vi "Delete Pulse.vi"(8 "error in (no error)":errorcluster, 10 "Shot":i32, 11 "Tree in":refnum<class "Tree.lvclass">) -> (0 "error out":errorcluster, 3 "Tree out":refnum<class "Tree.lvclass">)   [LabVIEW 2013, in "MDSplus.lvlib" / "Tree.lvclass"]
doc: "Delete a pulse file."
uses:
  <vilib>/MDSplus/Classes/Tree_Class/Tree.lvclass
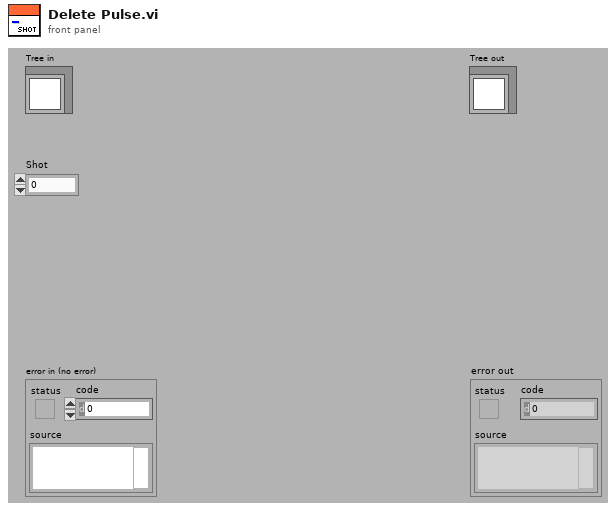
[diagram p1: front panel]
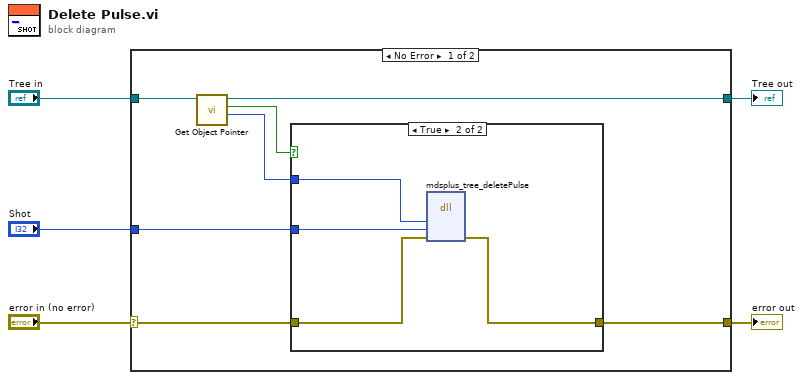
[diagram p0: block diagram]
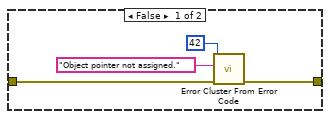
[diagram p2: hidden frame]
diagram:
  n1 = case shown="No Error" "error in (no error)" {
    selector: "error in (no error)" -> [w7 w22]
    tunnel: [w6 w22] -> w4
    tunnel: [w11 w21] -> w2
    tunnel: "Tree in" -> [w12 w21]
    tunnel: "Shot" -> [w10 _]
    frame No Error {
      n2 = call-dynamic "Get Object Pointer.vi"("Tree in"=w12) -> ("Object Pointer"=w8:i64, "Assigned object pointer?"=w9:bool, "Tree out"=w11:refnum<class "Tree.lvclass">)  [unwired: 8 in]
      n3 = case shown="True" w9 {
        tunnel: w10 -> [_ w17]
        tunnel: w8 -> [_ w20]
        tunnel: w7 -> [w14 w19]
        tunnel: [w13 w18] -> w6
        frame False {
          n4 = call <vilib>:"Error Cluster From Error Code.vi"("error in (no error)"=w14, "error message (\"\")"="Object pointer not assigned." ("error message (\"\")"), "error code (0)"=42) -> ("error out"=w13:errorcluster)  [unwired: 6 in]
        }
        frame True {
          n5 = dll-call lib="MDSobjectsLVShr" fn="mdsplus_tree_deletePulse"("lvTreePtr"=w20, "shotIn"=w17, "error"=w19) -> ("error"=w18:errorcluster)  [unwired: 6 in, 2 out]
        }
      }
    }
    frame Error {
    }
  }
  "error out" <- w4
  "Tree out" <- w2
